vi "Controller.vi"() -> ()   [LabVIEW 2018]
uses:
  support/dataTYPEDEF.ctl
  user32.dll
panel:
  in  "RemoveFromList":bool
  in  "AddToList":bool
  in  "Move":T1
  out "StatusBar":string
  out "Error Out":errorcluster {"code" format="%.0x"}
  in  "SetAngle":T2 {"Wrist" min=0 max=360 step=1; "Forearm" min=0 max=360 step=1; "Elbow" min=0 max=360 step=1; "Shoulder" min=0 max=360 step=1; "Waist" min=0 max=360 step=1}
  in  "MoveToPosition":bool
  in  "Name":string
  in  "Close":bool
  in  "Named Positions":i32(listbox)
  in  "Titlebar":bool
  in  "Color Theme":T3
  # "122/122/127"
  # "Angle"
  # "Move"
  # "Actions"
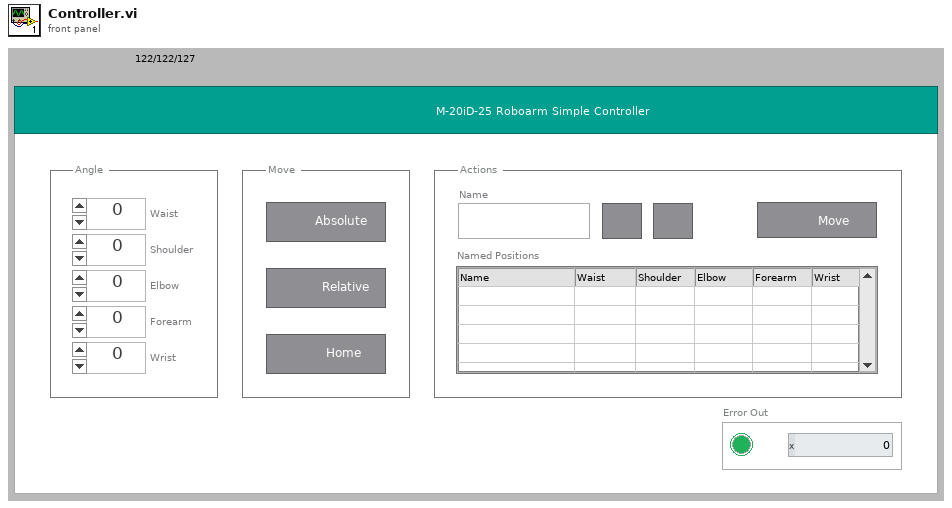
[diagram p1: front panel]
types:
  T1 = cluster{"Absolute":bool, "Relative":bool, "Home":bool}
  T2 = cluster{"Waist":i16, "Shoulder":i16, "Elbow":i16, "Forearm":i16, "Wrist":i16}
  T3 = cluster{"Theme color":u32, "Close button highlight color":u32}
  T4 = enum32{"Invalid", "Standard", "Closed", "Hidden", "Minimized", "Maximized"}
  T5 = enum32{"invalid app kind", "Development System", "Run Time System", "Student Edition", "Embedded LabVIEW", "Evaluation", "Custom"}
  T6 = cluster{"Close button highlight color":u32, "Close button highlight color":u32}
  T7 = cluster{"Close button highlight color":u32, "Close button highlight color":u32}[]
  T8 = typedef "dataTYPEDEF.ctl" = cluster{"angle[5]":i16[], "namedPositions[]":cluster{"name":string, "angle[5]":i16[]}[], "statuses":cluster{"messages":string[]}, "axis":refnum<k21>[], "currentPosition[5]":i16[]}
  T9 = cluster{"Core":cluster{"Current VI Reference":refnum<vi>, "Close Panel on Exit?":bool}, "data":T8}
  T10 = cluster{"Current VI Reference":refnum<vi>, "Close Panel on Exit?":bool}
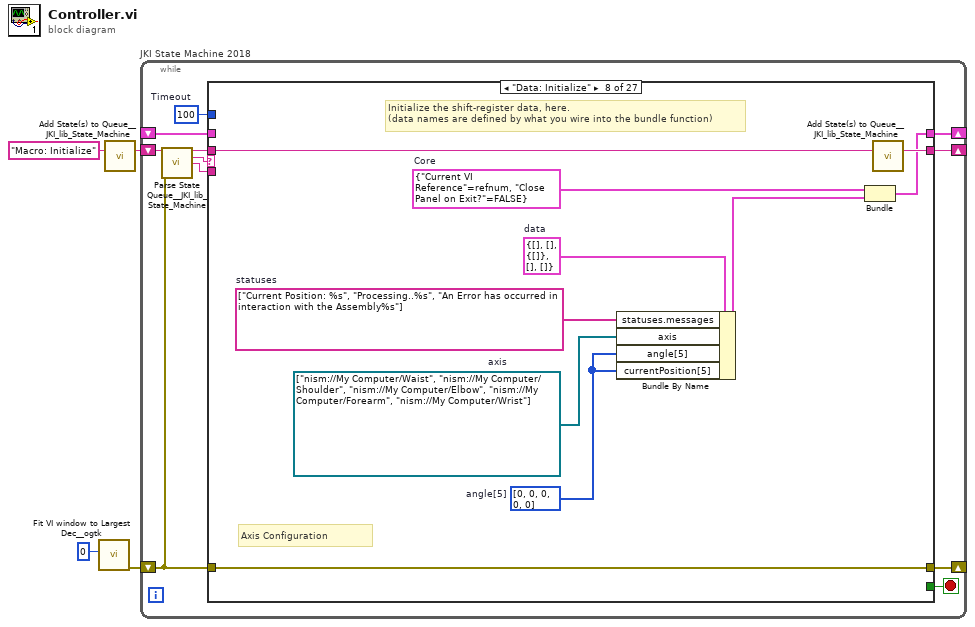
[diagram p0: block diagram]
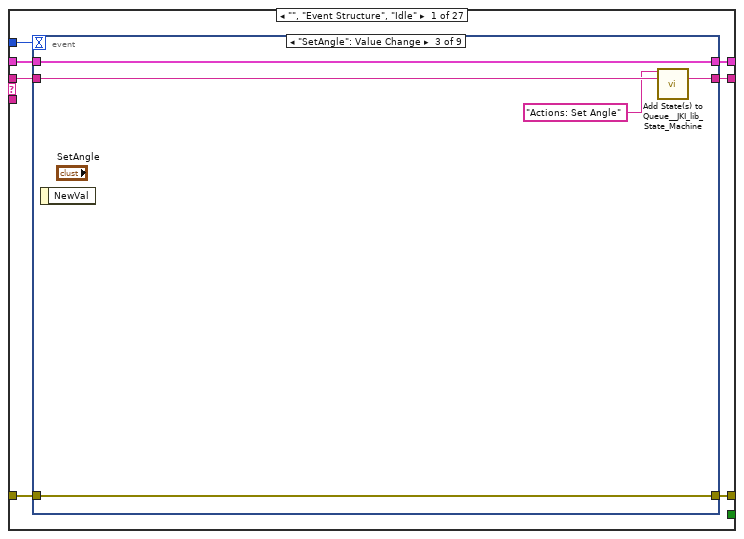
[diagram p2: hidden frame]
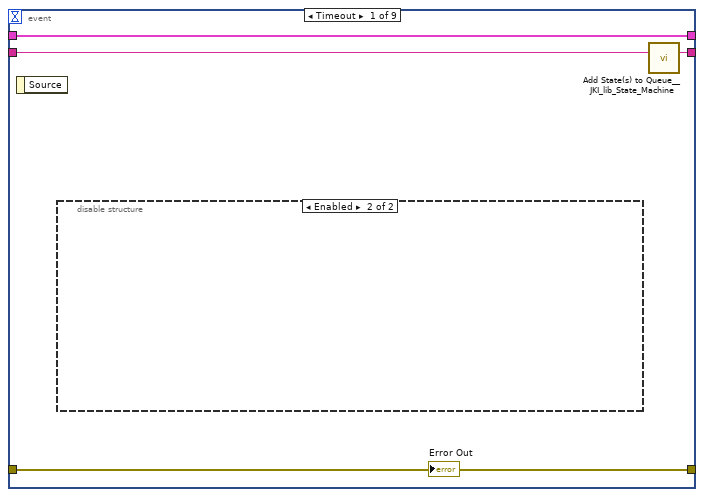
[diagram p3: hidden frame]
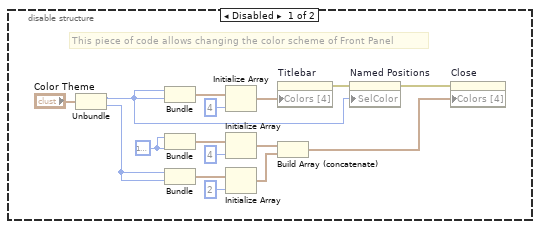
[diagram p4: hidden frame]
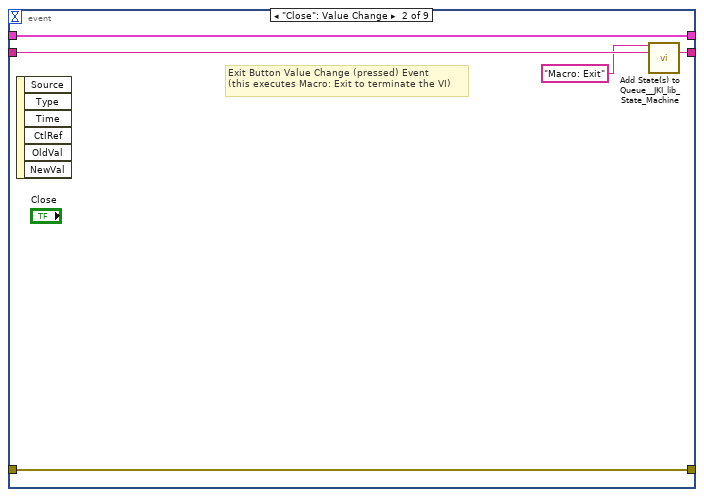
[diagram p5: hidden frame]
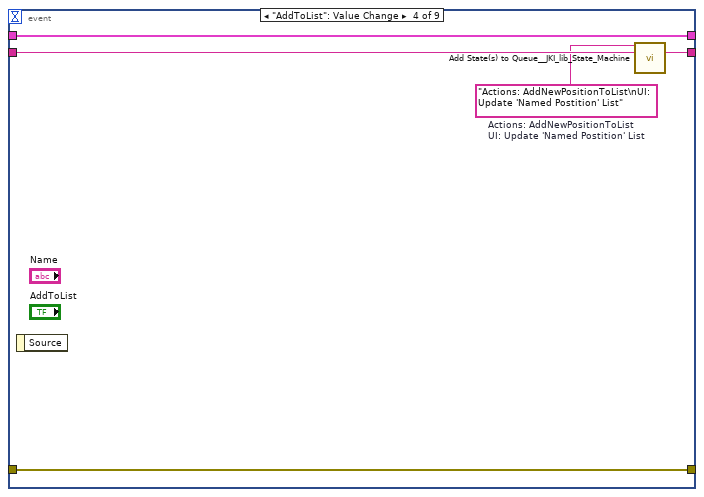
[diagram p6: hidden frame]
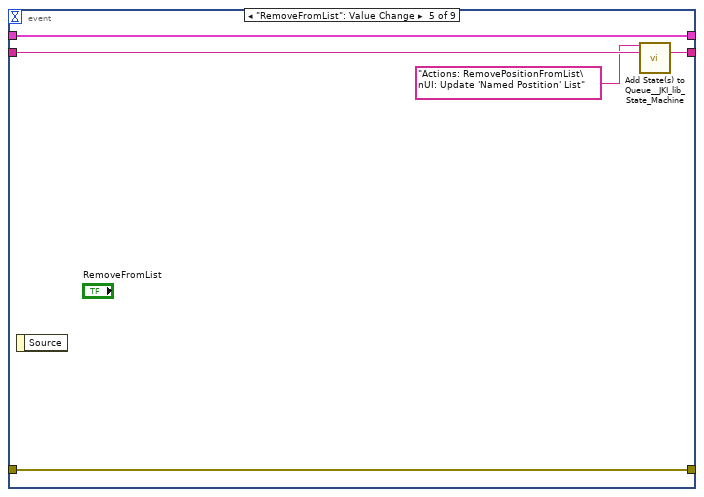
[diagram p7: hidden frame]
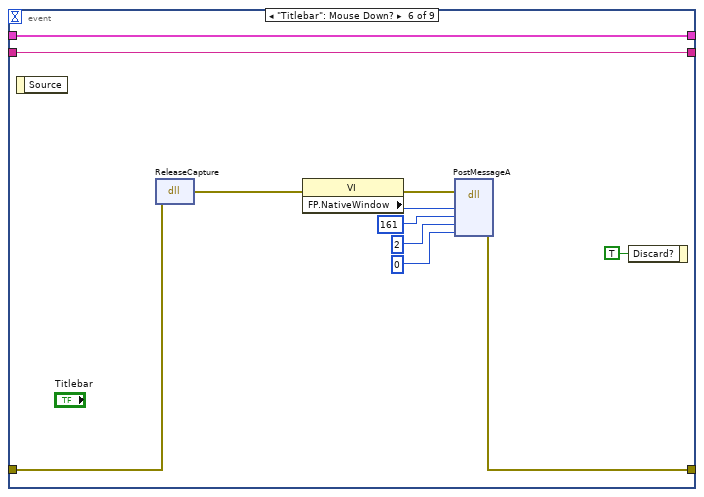
[diagram p8: hidden frame]
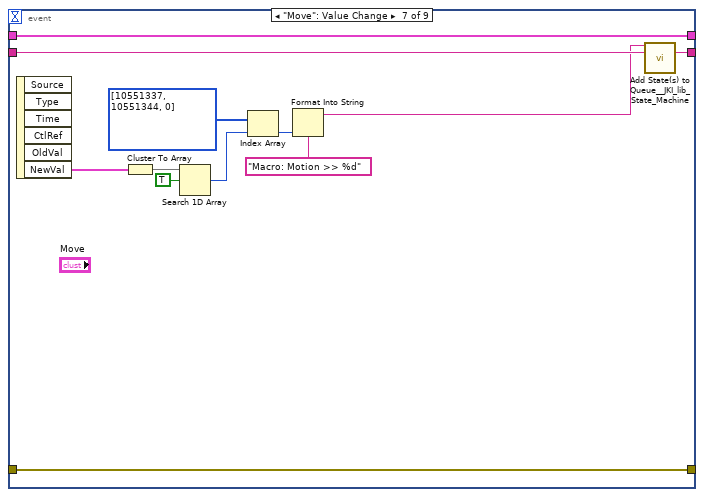
[diagram p9: hidden frame]
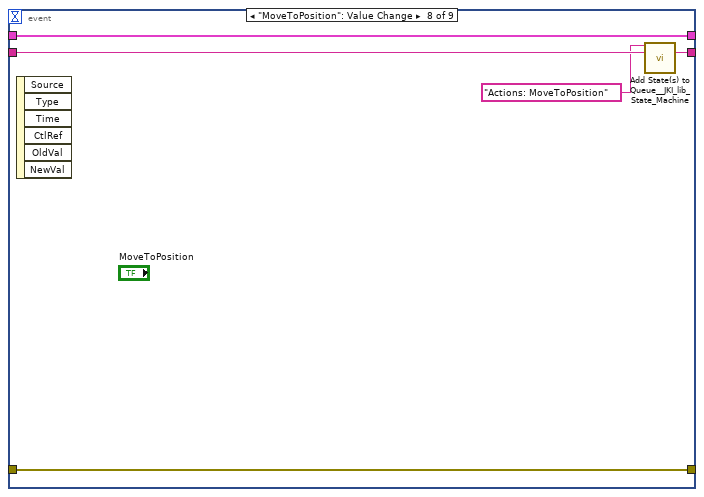
[diagram p10: hidden frame]
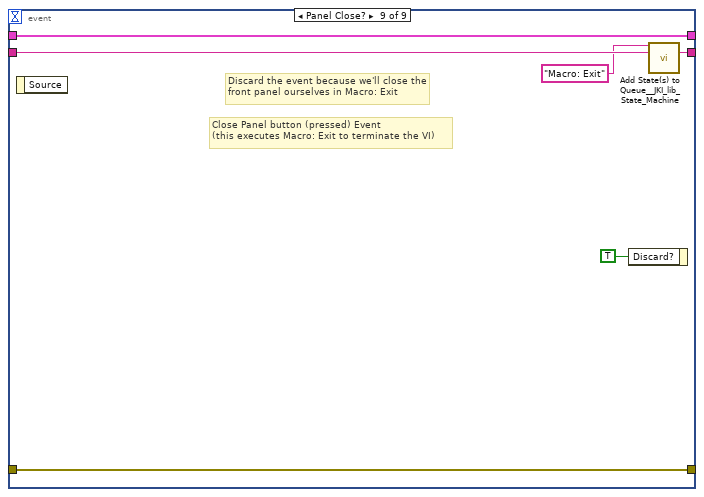
[diagram p11: hidden frame]
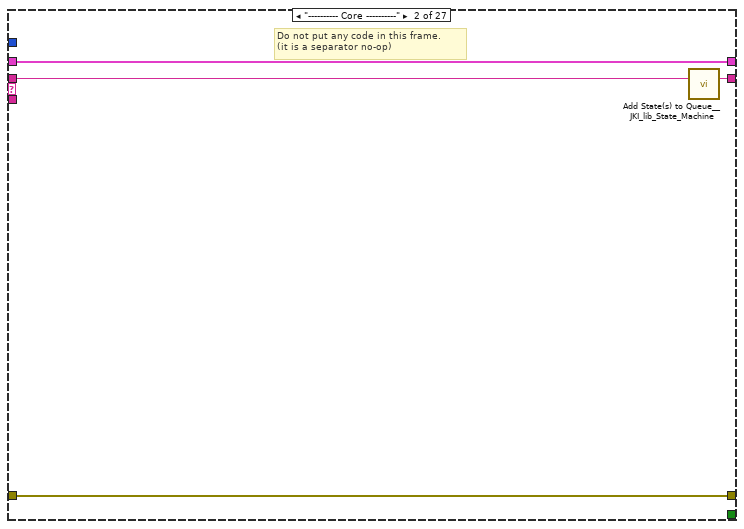
[diagram p12: hidden frame]
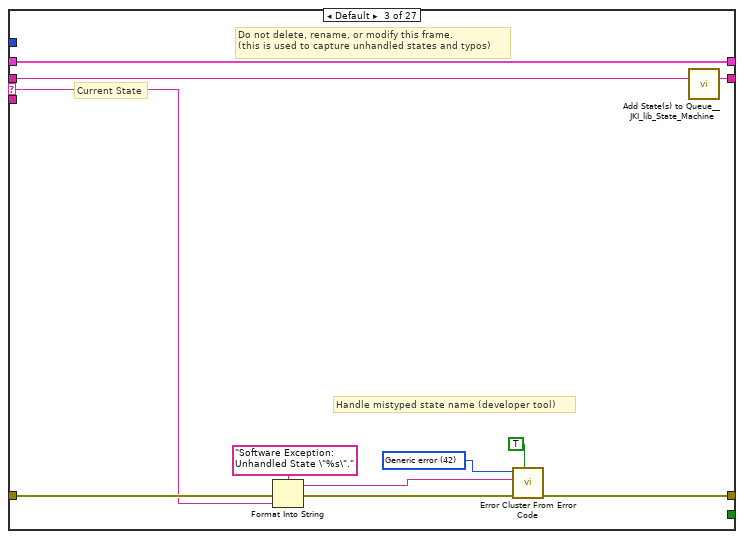
[diagram p13: hidden frame]
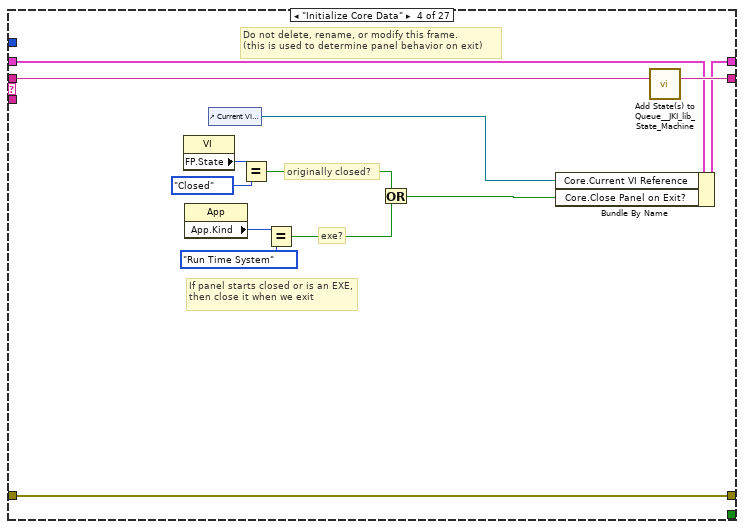
[diagram p14: hidden frame]
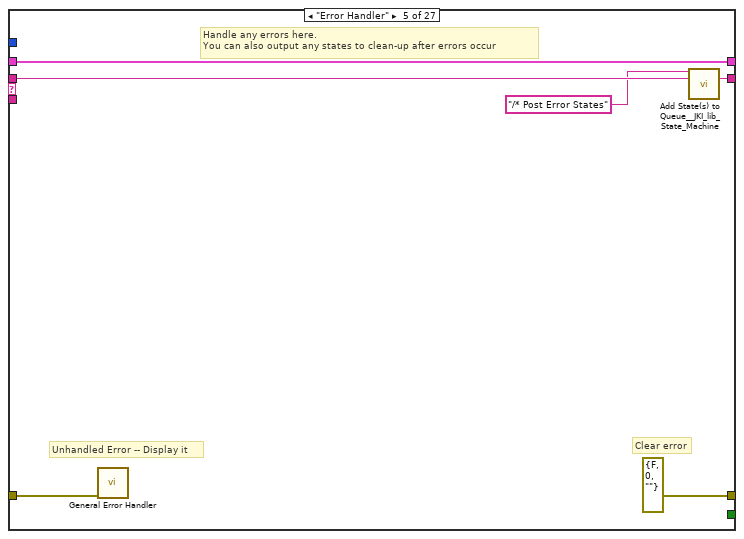
[diagram p15: hidden frame]
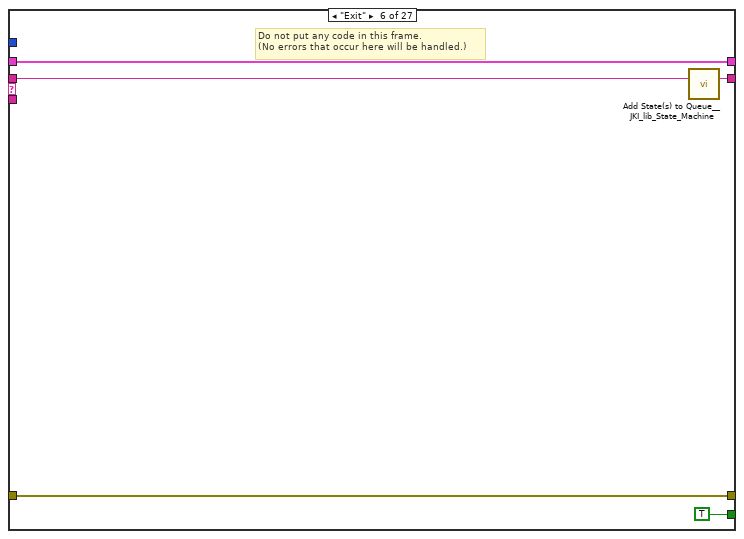
[diagram p16: hidden frame]
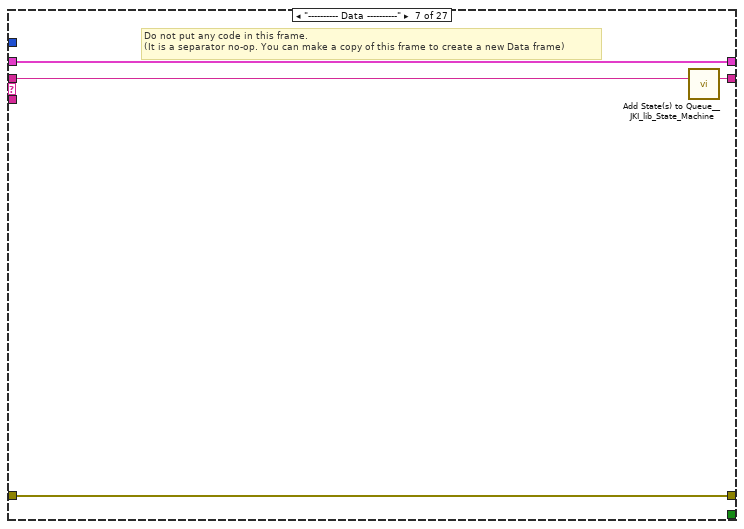
[diagram p17: hidden frame]
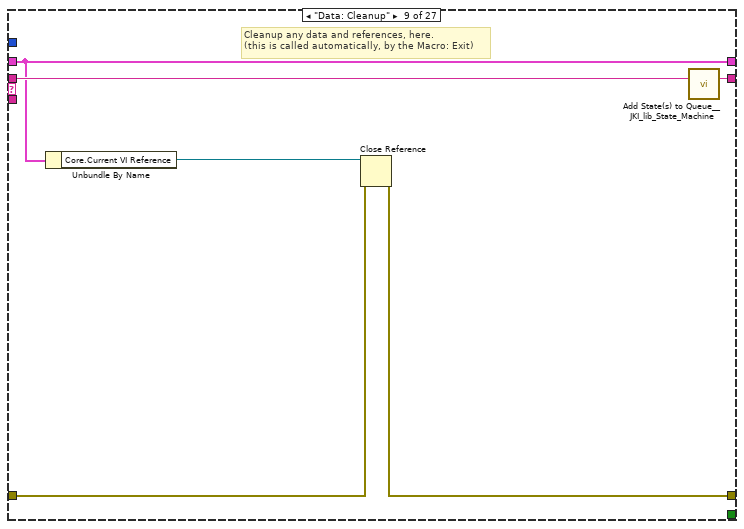
[diagram p18: hidden frame]
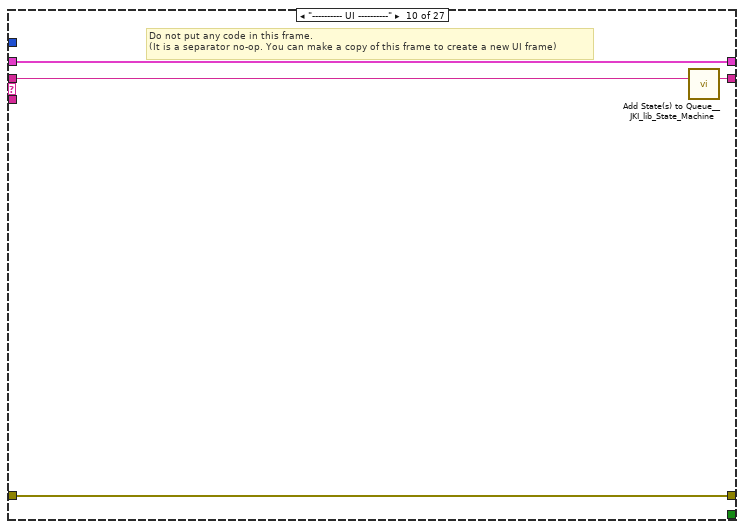
[diagram p19: hidden frame]
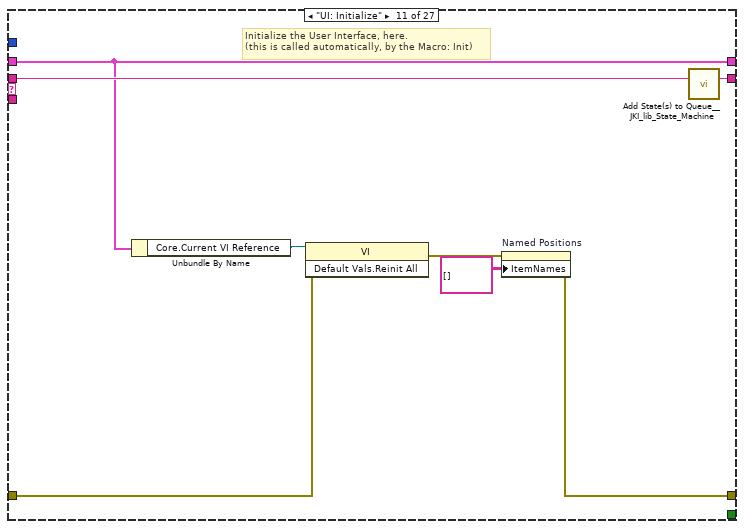
[diagram p20: hidden frame]
diagram:
  n1 = call <userlib>:"Fit VI window to Largest Dec__ogtk.vi"("border spacing (2 px)"=0) -> ("error out"=w1:errorcluster)  [unwired: 5 in, 1 out]
  n2 = call <vilib>:"Add State(s) to Queue__JKI_lib_State_Machine.vi"("State(s) in (\"\")"="Macro: Initialize") -> ("States Out"=w3:string)  [unwired: 14 in]
  n3 = while "JKI State Machine 2018" {
    shift-right: [w8] -> _
    shift-left: _ -> [w7]
    shift-right: [w11] -> _
    shift-left: w1 -> [w5]
    shift-right: [w10] -> _
    shift-left: w3 -> [w12]
    stop <- w9 stop-if-true
    w6 = 100  # Timeout
    n4 = call <vilib>:"Parse State Queue__JKI_lib_State_Machine.vi"("State Queue"=w12, "Error In (no error)"=w5) -> ("Remaining States"=w14:string, "Current State"=w15:string, "Arguments"=w13:string)  [unwired: 11 in]
    n5 = case shown="\"Data: Initialize\"" w15 {
      selector: w15 -> [_ _ w101 _ _ _ _ _ _ _ _ _ _ _ _ _ _ _ _ _ _ _ _ _ _ _ _]
      tunnel: w14 -> [w22 w100 w105 w124 w130 w135 w139 w149 w155 w159 w167 w173 w184 w256 w274 w278 w283 w294 w304 w308 w316 w342 w354 w363 w378 w398 w442]
      tunnel: w13 -> [_ _ _ _ _ _ _ _ _ _ _ w168 w178 _ w269 _ _ w291 _ _ _ _ _ _ _ w393 w440]
      tunnel: w7 -> [w20 w97 w103 w117 w127 w133 w136 _ w150 w156 w165 w171 w180 w252 w272 w275 w280 w292 w301 w305 w309 w335 w346 w360 w375 w380 w430]
      tunnel: [w19 w98 w107 w121 errorcluster {"status"=FALSE, "code"=0, "source"=""} ("error out") w132 w137 w146 w151 w157 w161 w169 w181 w251 w262 w276 w281 w285 w302 w306 w312 w338 w345 w358 w376 w387 w419] -> w11
      tunnel: w5 -> [w18 w98 w106 w121 w126 w132 w137 w146 w152 w157 w163 w170 w182 w250 w264 w276 w281 w290 w302 w306 w311 w337 w344 w359 w376 w388 w427]
      tunnel: [w21 w99 w104 w123 w129 w134 w138 w148 w154 w158 w166 w172 w183 w255 w273 w277 w282 w293 w303 w307 w315 w341 w353 w362 w377 w397 w441] -> w10
      tunnel: [_ _ _ _ _ TRUE _ _ _ _ _ _ _ _ _ _ _ _ _ _ _ _ _ _ _ _ _] -> w9
      tunnel: [w17 w97 w103 w122 w127 w133 w136 w147 w150 w156 w165 w171 w180 w252 w272 w275 w280 w292 w301 w305 w313 w336 w347 w361 w375 w381 w431] -> w8
      tunnel: w6 -> [w16 _ _ _ _ _ _ _ _ _ _ _ _ _ _ _ _ _ _ _ _ _ _ _ _ _ _]
      frame "", "Event Structure", "Idle" {
        n6 = event shown="[2] \"SetAngle\": Value Change" {
          selector: _ -> [_ _ _ _ _ _ _ _ _]
          dyn-events: _ -> [_ _ _ _ _ _ _ _ _]
          timeout: w16 -> [_ _ _ _ _ _ _ _ _]
          tunnel: w22 -> [w26 w47 w49 w56 w59 w71 w77 w89 w96]
          tunnel: [w25 w46 w50 w57 w60 w71 w76 w88 w95] -> w21
          tunnel: w20 -> [w24 w44 w52 w54 w61 w72 w78 w90 w93]
          tunnel: [w23 w45 w51 w53 w62 w63 w74 w87 w94] -> w19
          tunnel: w18 -> [w23 w45 w51 w53 w62 w64 w74 w87 w94]
          tunnel: [w24 w44 w52 w54 w61 w72 w78 w90 w93] -> w17
          event Timeout {
            n7 = event-data() -> ()  [unwired: 1 in, 1 out]
            n8 = disable-structure shown="Enabled" {
              frame Disabled {
                w30 = u32 16777216 ("Color Box")
                # "This piece of code allows changing the color scheme of Front Panel"
                n9 = Unbundle("Color Theme") -> ("Theme color"=w38:u32, "Close button highlight color"=w35:u32)
                n10 = Bundle("Theme color"=w38, "Theme color"=w38) -> (w32:cluster{"Theme color":u32, "Theme color":u32})  [unwired: 1 in]
                n11 = Bundle("Color Box"=w30, "Color Box"=w30) -> (w33:cluster{"Color Box":u32, "Color Box":u32})  [unwired: 1 in]
                n12 = Bundle("Close button highlight color"=w35, "Close button highlight color"=w35) -> (w34:T6)  [unwired: 1 in]
                n13 = Initialize Array(w32, 4 ("dimension size")) -> (w36:cluster{"Theme color":u32, "Theme color":u32}[])
                n14 = Initialize Array(w33, 4 ("dimension size")) -> (w40:cluster{"Color Box":u32, "Color Box":u32}[])
                n15 = Initialize Array(w34, 2 ("dimension size")) -> (w41:T7)
                n16 = property on="Titlebar" class="Bool (strict)"("Colors [4]"=w36) -> (error out=w37:errorcluster)  [unwired: 2 in, 1 out]
                n17 = Build Array (concatenate)(w40, w41) -> (w42:T7)
                n18 = property on="Named Positions" class="MCListbox (strict)"(error in=w37, "SelColor"=w38) -> (error out=w39:errorcluster)  [unwired: 1 in, 1 out]
                n19 = property on="Close" class="Bool"(error in=w39, "Colors [4]"=w42) -> ()  [unwired: 1 in, 2 out]
              }
              frame Enabled {
              }
            }
            n20 = call <vilib>:"Add State(s) to Queue__JKI_lib_State_Machine.vi"("State(s) in (\"\")"=w26) -> ("States Out"=w25:string)  [unwired: 14 in]
            "Error Out" <- w23
          }
          event "Close": Value Change {
            # "Exit Button Value Change (pressed) Event\n(this executes Macro: Exit to terminate the VI)"
            n21 = event-data() -> ()  [unwired: 1 in, 6 out]
            n22 = call <vilib>:"Add State(s) to Queue__JKI_lib_State_Machine.vi"("State(s) in Front (\"\")"="Macro: Exit", "State(s) in (\"\")"=w47) -> ("States Out"=w46:string)  [unwired: 13 in]
          }
          event "SetAngle": Value Change {
            n23 = event-data() -> ()  [unwired: 1 in, 1 out]
            n24 = call <vilib>:"Add State(s) to Queue__JKI_lib_State_Machine.vi"("State(s) in Front (\"\")"="Actions: Set Angle", "State(s) in (\"\")"=w49) -> ("States Out"=w50:string)  [unwired: 13 in]
          }
          event "AddToList": Value Change {
            w55 = "Actions: AddNewPositionToList\nUI: Update 'Named Postition' List"  # Actions: AddNewPositionToList UI: Update 'Named Postition' List
            n25 = event-data() -> ()  [unwired: 1 in, 1 out]
            n26 = call <vilib>:"Add State(s) to Queue__JKI_lib_State_Machine.vi"("State(s) in Front (\"\")"=w55, "State(s) in (\"\")"=w56) -> ("States Out"=w57:string)  [unwired: 13 in]
          }
          event "RemoveFromList": Value Change {
            n27 = event-data() -> ()  [unwired: 1 in, 1 out]
            n28 = call <vilib>:"Add State(s) to Queue__JKI_lib_State_Machine.vi"("State(s) in Front (\"\")"="Actions: RemovePositionFromList\nUI: Update 'Named Postition' List", "State(s) in (\"\")"=w59) -> ("States Out"=w60:string)  [unwired: 13 in]
          }
          event "Titlebar": Mouse Down? {
            n29 = event-data() -> ()  [unwired: 1 in, 1 out]
            n30 = dll-call lib="user32.dll" fn="ReleaseCapture"(error in=w64) -> (error out=w70:errorcluster)  [unwired: 3 in, 1 out]
            n31 = property class="VI"(error in=w70) -> (error out=w69:errorcluster, "FP.NativeWindow"=w68:u64)  [unwired: 1 in, 1 out]
            n32 = dll-call lib="user32.dll" fn="PostMessageA"(error in=w69, "hWnd"=w68, "Msg"=161, "wParam"=2, "lParam"=0) -> (error out=w63:errorcluster)  [unwired: 7 in, 1 out]
            n33 = event-data("Discard?"=TRUE) -> ()  [unwired: 1 in, 1 out]
          }
          event "Move": Value Change {
            w82 = i32[] [10551337, 10551344, 0] items=["BasePoint"=0, "Relative"=10551344, "Absolute"=10551337]
            n34 = event-data() -> ("NewVal"=w85:T1)  [unwired: 1 in, 5 out]
            n35 = Cluster To Array(cluster=w85) -> (array=w84:bool[])
            n36 = Search 1D Array(1D array=w84, element=TRUE) -> (index of element=w81:i32)  [unwired: 1 in]
            n37 = Index Array(array=w82, index=w81) -> (element=w80:i32)
            n38 = Format Into String(format string="Macro: Motion >> %d", w80) -> (resulting string=w75:string)  [unwired: 2 in, 1 out]
            n39 = call <vilib>:"Add State(s) to Queue__JKI_lib_State_Machine.vi"("State(s) in Front (\"\")"=w75, "State(s) in (\"\")"=w77) -> ("States Out"=w76:string)  [unwired: 13 in]
          }
          event "MoveToPosition": Value Change {
            n40 = event-data() -> ()  [unwired: 1 in, 6 out]
            n41 = call <vilib>:"Add State(s) to Queue__JKI_lib_State_Machine.vi"("State(s) in Front (\"\")"="Actions: MoveToPosition", "State(s) in (\"\")"=w89) -> ("States Out"=w88:string)  [unwired: 13 in]
          }
          event Panel Close? {
            # "Discard the event because we'll close the front panel ourselves in Macro: Exit"
            # "Close Panel button (pressed) Event\n(this executes Macro: Exit to terminate the VI)"
            n42 = event-data() -> ()  [unwired: 1 in, 1 out]
            n43 = event-data("Discard?"=TRUE) -> ()  [unwired: 1 in, 1 out]
            n44 = call <vilib>:"Add State(s) to Queue__JKI_lib_State_Machine.vi"("State(s) in Front (\"\")"="Macro: Exit", "State(s) in (\"\")"=w96) -> ("States Out"=w95:string)  [unwired: 13 in]
          }
        }
      }
      frame "---------- Core ----------" {
        # "Do not put any code in this frame.\n(it is a separator no-op)"
        n45 = call <vilib>:"Add State(s) to Queue__JKI_lib_State_Machine.vi"("State(s) in (\"\")"=w100) -> ("States Out"=w99:string)  [unwired: 14 in]
      }
      frame Default {
        w110 = 42 items=["No error", "Argument error", "Memory is full", "Out of zone", "End of file", "File already open", "Generic file I/O error", "File not found", "File permission error", "Disk is full", "Duplicate path", "Too many files open", "System feature not enabled", "Resource file not found", "Cannot add resource", "Resource not found", "Image not found", "Image memory error", "Pen does not exist", "Config type invalid", "Config token not found", "Config parse error", "Config memory error", "Bad external code format", "Bad external code offset", "External code not present", "Null window", "Destroy window error", "Null menu", "Print aborted", "Bad print record", "Print driver error", "Windows error during printing", "Memory error during printing", "Print dialog error", "Generic print error", "Invalid device refnum", "Device not found", "Device parameter error", "Device unit error", "Cannot open device", "Device call aborted", "Generic error", "Cancelled by user", "Object ID too low", "Object ID too high", "Object not in heap", "Unknown heap", "Unknown object (invalid DefProc)", "Unknown object (DefProc not in table)", "Message out of range", "Invalid (null) method", "Unknown message", "Manager call not supported", "Bad address", "Network operation in progress", "Network operation timed out", "Connection is busy", "Network attribute not supported", "Network error", "Address in use", "System out of memory", "Connection aborted", "Connection refused", "Not connected", "Already connected", "Connection closed", "Initialization error (interapplication manager)", "Bad occurrence", "Wait on unbound occurrence handler", "Occurrence queue overflow", "Datalog type conflict", "Unused", "Unrecognized type (interapplication manager)", "Memory corrupt", "Failed to make temporary DLL", "Old CIN version", "Drag socket not found", "Failed to load drop-object", "Failed to register OLE object", "Failed to release OLE object", "Format specifier type mismatch", "Unknown format specifier", "Too few format specifiers", "Too many format specifiers", "Scan failed", "Newer CIN version", "Error converting to variant", "Runtime menu error", "Password tampered", "Variant attribute not found", "Incompatible variant data type", "Event data is not available", "Event Store is not present", "Occurrence is not found", "Event Queue is not created", "Event info is not available", "Refnum passed is NULL", "Error retrieving Class GUID", "Error retrieving CoClass GUID", "Error retrieving TypeLib GUID.", "Bad built application magic bytes.", "Specific driver is different from the specific driver associated with the Logical Name.", "There is no session opened to the class driver.", "Max Error", "MAX - Error with config objects", "MAX - Error loading configuration", "MAX - Group not supported"]
        # "Current State"
        # "Do not delete, rename, or modify this frame.\n(this is used to capture unhandled states and typos)"
        # "Handle mistyped state name (developer tool)"
        n46 = Format Into String(format string="Software Exception: Unhandled State \"%s\"." ("message"), error in=w106, w101) -> (resulting string=w109:string, error out=w108:errorcluster)  [unwired: 1 in]
        n47 = call <vilib>:"Error Cluster From Error Code.vi"("show call chain? (False)"=TRUE, "error in (no error)"=w108, "error message (\"\")"=w109, "error code (0)"=w110) -> ("error out"=w107:errorcluster)  [unwired: 5 in]
        n48 = call <vilib>:"Add State(s) to Queue__JKI_lib_State_Machine.vi"("State(s) in (\"\")"=w105) -> ("States Out"=w104:string)  [unwired: 14 in]
      }
      frame "Initialize Core Data" {
        # "Do not delete, rename, or modify this frame.\n(this is used to determine panel behavior on exit)"
        # "originally closed?"
        # "exe?"
        # "If panel starts closed or is an EXE, then close it when we exit"
        n49 = property class="VI"() -> ("FP.State"=w114:T4)  [unwired: 2 in, 2 out]
        n50 = property class="App"() -> ("App.Kind"=w120:T5)  [unwired: 2 in, 2 out]
        n51 = control-ref of="Current VI Reference"() -> (w115:refnum<vi>)
        n52 = Equal?(x=w114, y=T4."Closed" ("Front Panel Window:State")) -> (x = y?=w112:bool)
        n53 = Equal?(x=w120, y=T5."Run Time System" ("Application:Kind")) -> (x = y?=w118:bool)
        n54 = Or(x=w112, y=w118) -> (x .or. y?=w116:bool)
        n55 = Bundle By Name(cluster=w117, "Core.Current VI Reference"=w115, "Core.Close Panel on Exit?"=w116) -> (w122:T9)
        n56 = call <vilib>:"Add State(s) to Queue__JKI_lib_State_Machine.vi"("State(s) in (\"\")"=w124) -> ("States Out"=w123:string)  [unwired: 14 in]
      }
      frame "Error Handler" {
        # "Unhandled Error -- Display it"
        # "Handle any errors here.\nYou can also output any states to clean-up after errors occur"
        # "Clear error"
        n57 = call <vilib>:"General Error Handler.vi"("error in (no error)"=w126) -> ()  [unwired: 10 in, 5 out]
        n58 = call <vilib>:"Add State(s) to Queue__JKI_lib_State_Machine.vi"("State(s) in Front (\"\")"="/* Post Error States", "State(s) in (\"\")"=w130) -> ("States Out"=w129:string)  [unwired: 13 in]
      }
      frame "Exit" {
        # "Do not put any code in this frame.\n(No errors that occur here will be handled.)"
        n59 = call <vilib>:"Add State(s) to Queue__JKI_lib_State_Machine.vi"("State(s) in (\"\")"=w135) -> ("States Out"=w134:string)  [unwired: 14 in]
      }
      frame "---------- Data ----------" {
        # "Do not put any code in this frame.\n(It is a separator no-op. You can make a copy of this frame to create a new Data frame)"
        n60 = call <vilib>:"Add State(s) to Queue__JKI_lib_State_Machine.vi"("State(s) in (\"\")"=w139) -> ("States Out"=w138:string)  [unwired: 14 in]
      }
      frame "Data: Initialize" {
        w140 = i16[] [0, 0, 0, 0, 0]  # angle[5]
        w141 = refnum<k21>[] ["nism://My Computer/Waist", "nism://My Computer/Shoulder", "nism://My Computer/Elbow", "nism://My Computer/Forearm", "nism://My Computer/Wrist"]  # axis
        w143 = string[] ["Current Position: %s", "Processing..%s", "An Error has occurred in interaction with the Assembly%s"]  # statuses
        w144 = T8 {"angle[5]"=[], "namedPositions[]"=[], "statuses"={"messages"=[]}, "axis"=[], "currentPosition[5]"=[]}  # data
        w145 = T10 {"Current VI Reference"=refnum, "Close Panel on Exit?"=FALSE}  # Core
        # "Axis Configuration"
        # "Initialize the shift-register data, here.\n(data names are defined by what you wire into the bundle function)"
        n61 = Bundle By Name(cluster=w144, "statuses.messages"=w143, "axis"=w141, "angle[5]"=w140, "currentPosition[5]"=w140) -> (w142:T8)
        n62 = Bundle("Core"=w145, "data"=w142) -> (w147:T9)  [unwired: 1 in]
        n63 = call <vilib>:"Add State(s) to Queue__JKI_lib_State_Machine.vi"("State(s) in (\"\")"=w149) -> ("States Out"=w148:string)  [unwired: 14 in]
      }
      frame "Data: Cleanup" {
        # "Cleanup any data and references, here.\n(this is called automatically, by the Macro: Exit)"
        n64 = Unbundle By Name(w150) -> ("Core.Current VI Reference"=w153:refnum<vi>)
        n65 = Close Reference(reference=w153, error in (no error)=w152) -> (error out=w151:errorcluster)
        n66 = call <vilib>:"Add State(s) to Queue__JKI_lib_State_Machine.vi"("State(s) in (\"\")"=w155) -> ("States Out"=w154:string)  [unwired: 14 in]
      }
      frame "---------- UI ----------" {
        # "Do not put any code in this frame.\n(It is a separator no-op. You can make a copy of this frame to create a new UI frame)"
        n67 = call <vilib>:"Add State(s) to Queue__JKI_lib_State_Machine.vi"("State(s) in (\"\")"=w159) -> ("States Out"=w158:string)  [unwired: 14 in]
      }
      frame "UI: Initialize" {
        # "Initialize the User Interface, here.\n(this is called automatically, by the Macro: Init)"
        n68 = Unbundle By Name(w165) -> ("Core.Current VI Reference"=w164:refnum<vi>)
        n69 = invoke class="VI" method="Default Vals.Reinit All"(reference=w164, error in=w163) -> (error out=w162:errorcluster)  [unwired: 1 in, 2 out]
        n70 = property on="Named Positions" class="MCListbox (strict)"(error in=w162, "ItemNames"=string[][] [] ("Item Names")) -> (error out=w161:errorcluster)  [unwired: 1 in, 1 out]
        n71 = call <vilib>:"Add State(s) to Queue__JKI_lib_State_Machine.vi"("State(s) in (\"\")"=w167) -> ("States Out"=w166:string)  [unwired: 14 in]
      }
      frame "UI: Cursor Set" {
        # "Argument"
        # "Set and Unset Cursor Busy.\n(Usage: \"UI: Cursor Set >> Busy|Idle\")"
        n72 = case shown="\"Busy\"" w168 {
          tunnel: w170 -> [w175 w177]
          tunnel: [w174 w176] -> w169
          frame "Idle", Default {
            n73 = call <vilib>:"Unset Busy.vi"("error in (no error)"=w175) -> ("error out"=w174:errorcluster)  [unwired: 10 in]
          }
          frame "Busy" {
            n74 = call <vilib>:"Set Busy.vi"("error in (no error)"=w177) -> ("error out"=w176:errorcluster)  [unwired: 9 in, 1 out]
          }
        }
        n75 = call <vilib>:"Add State(s) to Queue__JKI_lib_State_Machine.vi"("State(s) in (\"\")"=w173) -> ("States Out"=w172:string)  [unwired: 14 in]
      }
      frame "UI: Front Panel State" {
        # "Argument"
        # "Set Front Panel Open or Closed\n(Usage: \"UI: Front Panel State >> Open|Close\")"
        n76 = Unbundle By Name(w180) -> ("Core.Current VI Reference"=w179:refnum<vi>)
        n77 = case shown="\"Open\", \"Standard\", Default" w178 {
          tunnel: w182 -> [w190 w205 w216 w229 w242]
          tunnel: [w192 w206 w218 w231 w244] -> w181
          tunnel: w179 -> [w191 w203 w217 w230 w243]
          frame "Open", "Standard", Default {
            w185 = T4."Standard" ("State")
            n78 = property class="VI"(reference=w191, error in=w190) -> (reference out=w188:refnum<vi>, error out=w189:errorcluster, "FP.State"=w187:T4)
            n79 = Not Equal?(x=w187, y=w185) -> (x != y?=w186:bool)
            n80 = case shown="False" w186 {
              tunnel: [w196 w198] -> w192
              tunnel: w189 -> [w195 w198]
              tunnel: w188 -> [w194 _]
              tunnel: w185 -> [w193 _]
              frame True {
                n81 = invoke class="VI" method="FP.Open"(reference=w194, error in=w195, "Activate"=TRUE, "State"=w193) -> (error out=w196:errorcluster)  [unwired: 1 in, 4 out]
              }
              frame False {
              }
            }
          }
          frame "Close", "Closed" {
            n82 = property class="VI"(reference=w203, error in=w205) -> (reference out=w202:refnum<vi>, error out=w204:errorcluster, "FP.State"=w200:T4)
            n83 = Not Equal?(x=w200, y=T4."Closed" ("Front Panel Window:State")) -> (x != y?=w199:bool)
            n84 = case shown="True" w199 {
              tunnel: [w207 w210] -> w206
              tunnel: w204 -> [w207 w209]
              tunnel: w202 -> [_ w208]
              frame False {
              }
              frame True {
                n85 = invoke class="VI" method="FP.Close"(reference=w208, error in=w209) -> (error out=w210:errorcluster)  [unwired: 1 in, 2 out]
              }
            }
          }
          frame "Hidden", "Hide" {
            w211 = T4."Hidden" ("State")
            n86 = property class="VI"(reference=w217, error in=w216) -> (reference out=w214:refnum<vi>, error out=w215:errorcluster, "FP.State"=w213:T4)
            n87 = Not Equal?(x=w213, y=w211) -> (x != y?=w212:bool)
            n88 = case shown="True" w212 {
              tunnel: [w222 w223] -> w218
              tunnel: w215 -> [w221 w223]
              tunnel: w214 -> [w220 _]
              tunnel: w211 -> [w219 _]
              frame True {
                n89 = invoke class="VI" method="FP.Open"(reference=w220, error in=w221, "State"=w219) -> (error out=w222:errorcluster)  [unwired: 2 in, 4 out]
              }
              frame False {
              }
            }
          }
          frame "Minimize", "Minimized" {
            w224 = T4."Minimized" ("State")
            n90 = property class="VI"(reference=w230, error in=w229) -> (reference out=w227:refnum<vi>, error out=w228:errorcluster, "FP.State"=w226:T4)
            n91 = Not Equal?(x=w226, y=w224) -> (x != y?=w225:bool)
            n92 = case shown="True" w225 {
              tunnel: [w235 w236] -> w231
              tunnel: w228 -> [w234 w236]
              tunnel: w227 -> [w233 _]
              tunnel: w224 -> [w232 _]
              frame True {
                n93 = invoke class="VI" method="FP.Open"(reference=w233, error in=w234, "State"=w232) -> (error out=w235:errorcluster)  [unwired: 2 in, 4 out]
              }
              frame False {
              }
            }
          }
          frame "Maximize", "Maximized" {
            w237 = T4."Maximized" ("State")
            n94 = property class="VI"(reference=w243, error in=w242) -> (reference out=w240:refnum<vi>, error out=w241:errorcluster, "FP.State"=w239:T4)
            n95 = Not Equal?(x=w239, y=w237) -> (x != y?=w238:bool)
            n96 = case shown="True" w238 {
              tunnel: [w248 w249] -> w244
              tunnel: w241 -> [w247 w249]
              tunnel: w240 -> [w246 _]
              tunnel: w237 -> [w245 _]
              frame True {
                n97 = invoke class="VI" method="FP.Open"(reference=w246, error in=w247, "State"=w245) -> (error out=w248:errorcluster)  [unwired: 2 in, 4 out]
              }
              frame False {
              }
            }
          }
        }
        n98 = call <vilib>:"Add State(s) to Queue__JKI_lib_State_Machine.vi"("State(s) in (\"\")"=w184) -> ("States Out"=w183:string)  [unwired: 14 in]
      }
      frame "UI: Update 'Named Postition' List" {
        n99 = Unbundle By Name(w252) -> ("data.namedPositions[]"=w253:cluster{"name":string, "angle[5]":i16[]}[])
        n100 = for {
          tunnel: w253 -> [w261] mode=indexing
          tunnel: [w257] -> w254 mode=indexing
          n101 = Unbundle By Name(w261) -> ("name"=w259:string, "angle[5]"=w260:i16[])
          n102 = Number To Decimal String(number=w260) -> (decimal integer string=w258:string[])  [unwired: 1 in]
          n103 = Build Array (concatenate)(w259, w258) -> (w257:string[])
        }
        n104 = property on="Named Positions" class="MCListbox (strict)"(error in=w250, "ItemNames"=w254) -> (error out=w251:errorcluster)  [unwired: 1 in, 1 out]
        n105 = call <vilib>:"Add State(s) to Queue__JKI_lib_State_Machine.vi"("State(s) in (\"\")"=w256) -> ("States Out"=w255:string)  [unwired: 14 in]
      }
      frame "UI: UpdateStatusBar" {
        # "UI: UpdateStatusBar >> 1,"
        n106 = Unbundle By Name(w272) -> ("data.statuses.messages"=w271:string[])
        n107 = Scan From String(format string="%d, %[0-9 ,.]", input string=w269, error in=w264) -> (error out=w263:errorcluster, output 1=w267:i32, output 2=w266:string)  [unwired: 3 in, 2 out]
        n108 = Index Array(array=w271, index=w267) -> (element=w270:string)
        n109 = Format Into String(format string=w270, error in=w263, w266) -> (resulting string=→"StatusBar":string, error out=w262:errorcluster)  [unwired: 1 in]
        n110 = call <vilib>:"Add State(s) to Queue__JKI_lib_State_Machine.vi"("State(s) in (\"\")"=w274) -> ("States Out"=w273:string)  [unwired: 14 in]
      }
      frame "---------- Macro ----------" {
        # "Do not put any code in this frame.\n(It is a separator no-op. You can make a copy of this frame to create a new Macro frame)"
        n111 = call <vilib>:"Add State(s) to Queue__JKI_lib_State_Machine.vi"("State(s) in (\"\")"=w278) -> ("States Out"=w277:string)  [unwired: 14 in]
      }
      frame "Macro: Initialize" {
        w279 = "Data: Initialize\nInitialize Core Data\nUI: Initialize\nUI: Front Panel State >> Open"  # Data: Initialize Initialize Core Data UI: Initialize UI: Front Panel State >> Open
        # "Initialization Macro\n(This is called once, when the VI starts)"
        n112 = call <vilib>:"Add State(s) to Queue__JKI_lib_State_Machine.vi"("State(s) in Front (\"\")"=w279, "State(s) in (\"\")"=w283) -> ("States Out"=w282:string)  [unwired: 13 in]
      }
      frame "Macro: Motion" {
        w286 = "UI: Cursor Set >> Busy\nUI: UpdateStatusBar >> 1,.\nMotion: Move >> %d\nActions: Set Angle\nUI: Cursor Set >> Idle"  # UI: Cursor Set >> Busy UI: UpdateStatusBar >> 1,. Motion: Move >> %d Actions: Set Angle UI: Cursor Set >> Idle
        n113 = Scan From String(format string="%d", input string=w291, error in=w290) -> (error out=w288:errorcluster, output 1=w287:i32)  [unwired: 2 in, 2 out]
        n114 = Format Into String(format string=w286, error in=w288, w287) -> (resulting string=w284:string, error out=w285:errorcluster)  [unwired: 1 in]
        n115 = call <vilib>:"Add State(s) to Queue__JKI_lib_State_Machine.vi"("State(s) in Front (\"\")"=w284, "State(s) in (\"\")"=w294) -> ("States Out"=w293:string)  [unwired: 13 in]
      }
      frame "Macro: Exit" {
        # "Exit Macro\n(This is called once, when the VI exits)"
        n116 = Unbundle By Name(w301) -> ("Core.Close Panel on Exit?"=w300:bool)
        n117 = Select(t="UI: Front Panel State >> Close", s=w300, f="") -> (s? t:f=w297:string)
        n118 = call <vilib>:"Add State(s) to Queue__JKI_lib_State_Machine.vi"("State(s) in (\"\")"=w297, "State(s) at Back (\"\")"="Data: Cleanup\nExit") -> ("States Out"=w295:string)  [unwired: 13 in]
        n119 = call <vilib>:"Add State(s) to Queue__JKI_lib_State_Machine.vi"("State(s) in Front (\"\")"=w295, "State(s) in (\"\")"=w304) -> ("States Out"=w303:string)  [unwired: 13 in]
      }
      frame "---------- Actions ----------" {
        # "Template Separator\n(You can make a copy of, or modify, this frame)"
        n120 = call <vilib>:"Add State(s) to Queue__JKI_lib_State_Machine.vi"("State(s) in (\"\")"=w308) -> ("States Out"=w307:string)  [unwired: 14 in]
      }
      frame "Actions: MoveToPosition" {
        n121 = case shown="Default" "Named Positions" {
          selector: "Named Positions" -> [_ w322]
          tunnel: ["" w332] -> w314
          tunnel: [w317 w320] -> w313
          tunnel: [w318 w325] -> w312
          tunnel: w311 -> [w318 w324]
          tunnel: w309 -> [w317 w321]
          frame -1 {
          }
          frame Default {
            w333 = 10551337 items=["BasePoint"=0, "Relative"=10551344, "Absolute"=10551337] ("line move mode")
            n122 = property on="Named Positions" class="MCListbox (strict)"(error in=w324) -> (error out=w325:errorcluster, "ItemNames"=w331:string[][])  [unwired: 1 in, 1 out]
            n123 = Index Array(array=w331, index (row)=w322) -> (element=w330:string[])  [unwired: 1 in]
            n124 = Delete From Array(array=w330, length=1, index=0) -> (array with subset deleted=w327:string[])  [unwired: 1 out]
            n125 = Decimal String To Number(string=w327, default (0L)=i16 0 ("default (0 I32)")) -> (number=w323:i16[])  [unwired: 1 in, 1 out]
            n126 = Bundle By Name(cluster=w321, "data.angle[5]"=w323) -> (w320:T9)
            n127 = Format Into String(format string="Macro: Motion >> %d", w333) -> (resulting string=w332:string)  [unwired: 2 in, 1 out]
          }
        }
        n128 = call <vilib>:"Add State(s) to Queue__JKI_lib_State_Machine.vi"("State(s) in Front (\"\")"=w314, "State(s) in (\"\")"=w316) -> ("States Out"=w315:string)  [unwired: 13 in]
      }
      frame "Actions: Set Angle" {
        n129 = property on="SetAngle" class="Clust (strict)"(error in=w337) -> (error out=w338:errorcluster, "Value"=w340:T2)  [unwired: 1 in, 1 out]
        n130 = Cluster To Array(cluster=w340) -> (array=w339:i16[])
        n131 = Bundle By Name(cluster=w335, "data.angle[5]"=w339) -> (w336:T9)
        n132 = call <vilib>:"Add State(s) to Queue__JKI_lib_State_Machine.vi"("State(s) in (\"\")"=w342) -> ("States Out"=w341:string)  [unwired: 14 in]
      }
      frame "Actions: AddNewPositionToList" {
        n133 = Unbundle By Name(w346) -> ("data.namedPositions[]"=w352:cluster{"name":string, "angle[5]":i16[]}[], "data.angle[5]"=w349:i16[])
        n134 = property on="Name" class="Str"(error in=w344) -> (error out=w345:errorcluster, "Value"=w343:string)  [unwired: 1 in, 1 out]
        n135 = Bundle By Name(cluster=cluster{"name":string, "Angle[5]":i16[]} {"name"="", "Angle[5]"=[]} ("new element/subarray"), "Angle[5]"=w349, "name"=w343) -> (w348:cluster{"name":string, "Angle[5]":i16[]})
        n136 = Insert Into Array(array=w352, new element=w348) -> (w351:cluster{"name":string, "angle[5]":i16[]}[])  [unwired: 1 in]
        n137 = Bundle By Name(cluster=w346, "data.namedPositions[]"=w351) -> (w347:T9)
        n138 = call <vilib>:"Add State(s) to Queue__JKI_lib_State_Machine.vi"("State(s) in (\"\")"=w354) -> ("States Out"=w353:string)  [unwired: 14 in]
      }
      frame "Actions: RemovePositionFromList" {
        n139 = Unbundle By Name(w360) -> ("data.namedPositions[]"=w357:cluster{"name":string, "angle[5]":i16[]}[])
        n140 = property on="Named Positions" class="MCListbox (strict)"(error in=w359) -> (error out=w358:errorcluster, "Value"=w355:i32)  [unwired: 1 in, 1 out]
        n141 = Array Size(array=w357) -> (size(s)=w356:i32)
        n142 = case shown="Default" w356 {
          selector: w356 -> [_ w366]
          tunnel: [w364 w374] -> w361
          tunnel: w360 -> [w364 w373]
          tunnel: w357 -> [_ w371]
          tunnel: w355 -> [_ w369]
          frame 0 {
          }
          frame Default {
            n143 = Less Than 0?(x=w369) -> (x < 0?=w370:bool)
            n144 = Decrement(x=w366) -> (x-1=w365:i32)
            n145 = Select(t=w365, s=w370, f=w369) -> (s? t:f=w368:i32)
            n146 = Delete From Array(array=w371, length=1, index=w368) -> (array with subset deleted=w372:cluster{"name":string, "angle[5]":i16[]}[])  [unwired: 1 out]
            n147 = Bundle By Name(cluster=w373, "data.namedPositions[]"=w372) -> (w374:T9)
          }
        }
        n148 = call <vilib>:"Add State(s) to Queue__JKI_lib_State_Machine.vi"("State(s) in (\"\")"=w363) -> ("States Out"=w362:string)  [unwired: 14 in]
      }
      frame "---------- Motion ----------" {
        # "Template Separator\n(You can make a copy of, or modify, this frame)"
        n149 = call <vilib>:"Add State(s) to Queue__JKI_lib_State_Machine.vi"("State(s) in (\"\")"=w378) -> ("States Out"=w377:string)  [unwired: 14 in]
      }
      frame "Motion: Move" {
        w389 = 10551337 items=["Relative"=10551344, "Absolute"=10551337, "Relative To Capture"=10551345, "Velocity"=10551346, "Polyline"=11600101] ("line move mode")
        w394 = i16[] [0, 0, 0, 0, 0]  # Home position
        n150 = Unbundle By Name(w380) -> ("data.axis"=w396:refnum<k21>[], "data.angle[5]"=w395:i16[])
        n151 = Scan From String(format string="%d", input string=w393) -> (output 1=w391:i32)  [unwired: 3 in, 3 out]
        n152 = Not Equal To 0?(x=w391) -> (x != 0?=w390:bool)
        n153 = Select(t=w395, s=w390, f=w394) -> (s? t:f=w379:i16[])
        n154 = Select(t=w391, s=w390, f=w389) -> (s? t:f=w386:i32)
        n155 = for {
          tunnel: w396 -> [w413] mode=indexing
          shift-right: [w402] -> w387
          shift-left: w388 -> [w414]
          tunnel: w379 -> [w412] mode=indexing
          tunnel: w386 -> [w411]
          shift-right: [w403] -> w383
          shift-left: i16 0 -> [w405]
          i -> [w406]
          n156 = To Double Precision Float(number=w412) -> (double precision float=w410:dbl)
          n157 = call "commonMotionMove.vi"("timeout"=5000.0, "line move mode"=w411, "error in"=w414, "velocity"=3000.0, "position"=w410, "resource"=w413) -> ("error out"=w402:errorcluster, "timed out?"=w399:bool)  [unwired: 3 in, 1 out]
          n158 = Unbundle By Name(w402) -> ("status"=w401:bool)
          n159 = Or(x=w399, y=w401) -> (x .or. y?=w400:bool)
          n160 = Boolean To (0,1)(Boolean=w400) -> (0, 1=w407:i16)
          n161 = Logical Shift(y=w406, x=w407) -> (x << y=w404:i16)
          n162 = Add(x=w405, y=w404) -> (x+y=w403:i16)
        }
        n163 = Bundle By Name(cluster=w380, "data.angle[5]"=w379) -> (w381:T9)
        n164 = Format Into String(format string="Motion: UpdatePosition >> %d,%d", w386, w383) -> (resulting string=w382:string)  [unwired: 2 in, 1 out]
        n165 = call <vilib>:"Add State(s) to Queue__JKI_lib_State_Machine.vi"("State(s) in Front (\"\")"=w382, "State(s) in (\"\")"=w398) -> ("States Out"=w397:string)  [unwired: 13 in]
      }
      frame "Motion: UpdatePosition" {
        n166 = Unbundle By Name(w430) -> ("data.angle[5]"=w436:i16[], "data.currentPosition[5]"=w435:i16[])
        n167 = Scan From String(format string="%d,%d", input string=w440, error in=w427) -> (error out=w426:errorcluster, output 1=w437:i32, output 2=w432:i32)  [unwired: 3 in, 2 out]
        n168 = case shown="Default" w437 {
          tunnel: w436 -> [w452 w455]
          tunnel: w435 -> [w451 w453]
          tunnel: [w452 w454] -> w433
          tunnel: [w451 w453] -> w434
          frame Default {
          }
          frame 10551344 {
            # "Relative"
            n169 = Add(x=w455, y=w453) -> (x+y=w454:i16[])
          }
        }
        n170 = for {
          tunnel: w434 -> [w448] mode=indexing
          tunnel: w433 -> [w447] mode=indexing
          tunnel: w432 -> [w450]
          tunnel: [w446] -> w425 mode=indexing
          tunnel: [w445] -> w429 mode=indexing
          i -> [w444]
          n171 = expression code="x*(-1)"(w444) -> (w443:i32)
          n172 = Logical Shift(y=w443, x=w450) -> (x << y=w449:i32)
          n173 = Equal To 0?(x=w449) -> (x = 0?=w445:bool)
          n174 = Select(t=w447, s=w445, f=w448) -> (s? t:f=w446:i16)
        }
        n175 = And Array Elements(Boolean array=w429) -> (logical AND=w416:bool)
        n176 = Bundle By Name(cluster=w430, "data.currentPosition[5]"=w425) -> (w431:T9)
        n177 = Index Array(array=w425) -> (element #1=w424:i16, element #2=w423:i16, element #3=w422:i16, element #4=w421:i16, element #5=w420:i16)  [unwired: 5 in]
        n178 = Not(x=w416) -> (.not. x?=w415:bool)
        n179 = Format Into String(format string="UI: UpdateStatusBar >> 0,%d, %d, %d, %d, %d", error in=w426, w424, w423, w422, w421, w420) -> (resulting string=w417:string, error out=w419:errorcluster)  [unwired: 1 in]
        n180 = Select(t="UI: UpdateStatusBar >> 2,." ("format string"), s=w415, f=w417) -> (s? t:f=w418:string)
        n181 = call <vilib>:"Add State(s) to Queue__JKI_lib_State_Machine.vi"("State(s) in Front (\"\")"=w418, "State(s) in (\"\")"=w442) -> ("States Out"=w441:string)  [unwired: 13 in]
      }
    }
  }
